vi "CLD 8 CSV file commands utility Exercise.vi"(8 "Fehler (Eingang)":T2) -> (0 "Fehler (Ausgang)":T2, 3 "Befehls-Ausgangs-Array":T1[](array[typedef]))   [LabVIEW 2009]
doc: "CLD-Übung 8"
uses:
  CLD 8 Data Cluster.ctl
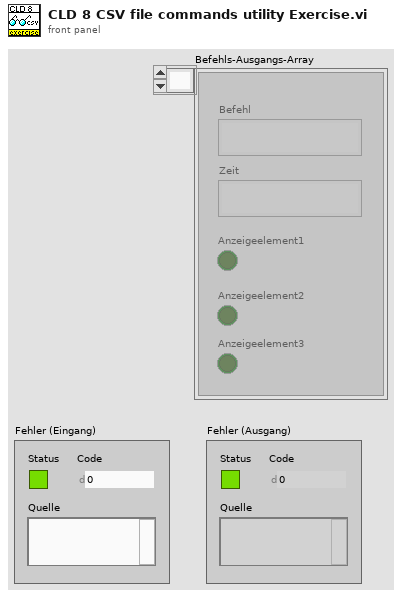
[diagram p1: front panel]
types:
  T1 = typedef "CLD 8 Data Cluster.ctl" = cluster{"Befehl":string, "Zeit":string, "Anzeigeelement1":bool, "Anzeigeelement2":bool, "Anzeigeelement3":bool}
  T2 = cluster{"Status":bool, "Code":i32, "Quelle":string}
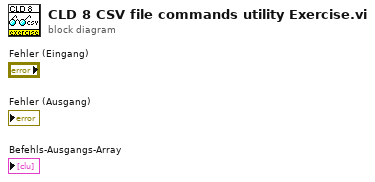
[diagram p0: block diagram]
diagram:
